vi "Create Tiger.vi"() -> (3 "output cluster":refnum<class "Tiger.lvclass">)   [LabVIEW 2018, in "Tiger.lvclass"]
uses:
  Tiger.lvclass
  animal/Animal.lvclass
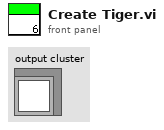
[diagram p1: front panel]
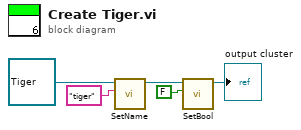
[diagram p0: block diagram]
diagram:
  n1 = call "SetName.vi"("Name"="tiger", "Animal in"=refnum<class "Tiger.lvclass"> refnum ("Tiger.lvclass")) -> ("Animal out"=w3:refnum<class "Tiger.lvclass">)  [unwired: 8 in, 1 out]
  n2 = call "SetBool.vi"("Bool"=FALSE, "Animal in"=w3) -> ("Animal out"=→"output cluster":refnum<class "Tiger.lvclass">)  [unwired: 8 in, 1 out]
